vi "Obtain-Gserver-Queue.vi"() -> (6 "Gserver Queue":refnum<queue>)   [LabVIEW 2020]
doc: "Obtain a queue for Gserver\nThis Queue is primary intended to be used to post Gviewer Queries"
uses:
  controls/Typedef_Gviewer-Query.ctl
  controls/Typedef_QueryType.ctl
  Gserver.lvclass
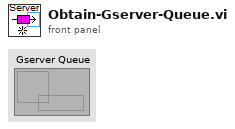
[diagram p1: front panel]
types:
  T1 = typedef "Sgraph_lib_V1.lvlib/Gserver.lvclass/Typedef_Gviewer-Query.ctl" = cluster{"Query_type":T2, "data":variant, "Source":string, "Time Stamp":timestamp}
  T2 = typedef "Sgraph_lib_V1.lvlib/Gserver.lvclass/Typedef_QueryType.ctl" = enum16{"Subscribe", "DataRequest", "RequestAllTags", "RequestIniPath", "FAMMstarted", "SetClientOptions", "GviewerUpdate", "OpenNewGraph", "CloseClient", "CloseAllClients", "Close Gserver", "OpenMemoryMap", "MeMapDataRequest", "MeMapDataResponse", "OpenDBeditor", "CheckDBeditorRunning", "StoppedDBeditor", "SaveDB_TAGpropRecord", "ConfirmDB_TAGpropSave", "GetXconstraints"}
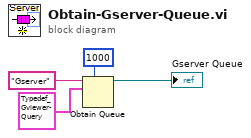
[diagram p0: block diagram]
diagram:
  n1 = Obtain Queue(max queue size (-1, unlimited)=1000, name (unnamed)="Gserver", element data type=T1 {"Query_type"=enum."DataRequest", "data"=variant, "Source"="", "Time Stamp"=timestamp(0 s since 1904-01-01)} ("Query")) -> (queue out=→"Gserver Queue":refnum<queue>)  [unwired: 2 in, 2 out]
